vi "alicat gas monitor.vi"() -> ()   [LabVIEW 2010]
uses:
  <vilib>/Utility/file.llb/Write To Spreadsheet File (DBL).vi
panel:
  out "error out":errorcluster
  in  "Path":path
  out "Alicat gas flow monitor":cluster{dbl, dbl}[](graph)
  out "Pressure (inH2O)":dbl
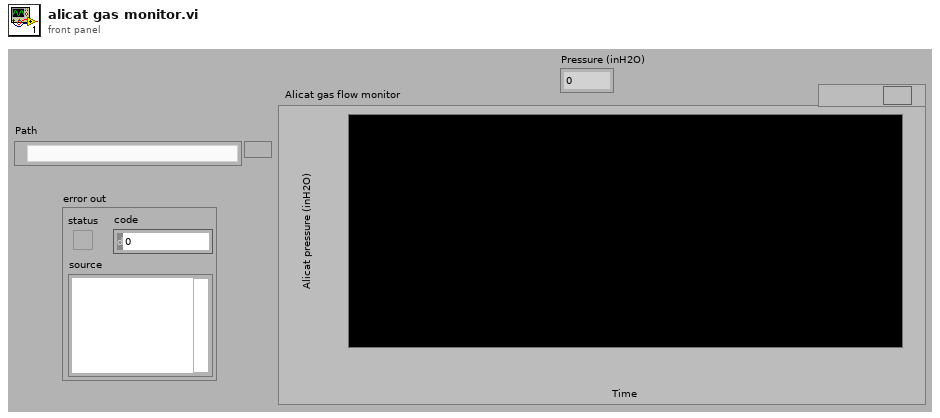
[diagram p1: front panel]
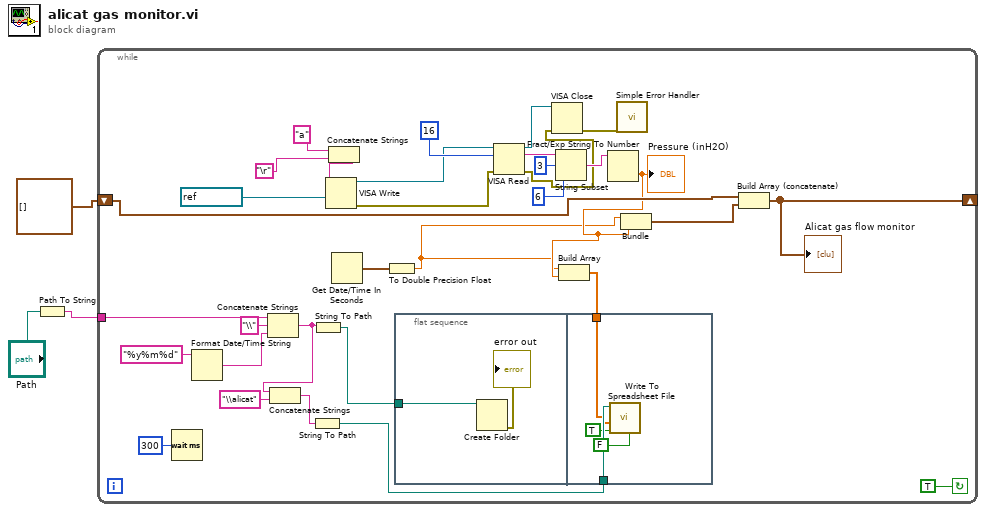
[diagram p0: block diagram]
diagram:
  n1 = Path To String(path="Path") -> (string=w1:string)
  n2 = while {
    shift-right: [w19] -> _
    shift-left: cluster{dbl, dbl}[] [] -> [w20]
    tunnel: w1 -> [w17]
    stop <- TRUE continue-if-true
    n3 = Wait (ms)(milliseconds to wait=u32 300) -> ()  [unwired: 1 out]
    n4 = Format Date/Time String(time format string (%c)="%y%m%d") -> (date/time string=w15:string)  [unwired: 2 in]
    n5 = Concatenate Strings(w17, "\\" ("string"), w15) -> (w12:string)
    n6 = Concatenate Strings(w12, "\\alicat" ("string")) -> (w11:string)
    n7 = String To Path(string=w11) -> (path=w10:path)
    n8 = String To Path(string=w12) -> (path=w14:path)
    n9 = Concatenate Strings("a" ("string"), "\r") -> (w34:string)
    n10 = VISA Write(VISA resource name=refnum<visa-resource-name> "COM6", write buffer=w34) -> (VISA resource name out=w29:refnum<visa-resource-name>, error out=w30:errorcluster)  [unwired: 1 in, 1 out]
    n11 = Get Date/Time In Seconds() -> (seconds since 1Jan1904=w22:timestamp)
    n12 = To Double Precision Float(number=w22) -> (double precision float=w8:dbl)
    n13 = flat-sequence {
      tunnel: w14 -> [w37]
      tunnel: w10 -> [w41]
      tunnel: w7 -> [w38]
      frame #0 {
        n14 = Create Folder(path (use dialog)=w37) -> (error out=→"error out":errorcluster)  [unwired: 2 in, 2 out]
      }
      frame #1 {
        n15 = call-poly <vilib>:"Write To Spreadsheet File.vi"("transpose? (no:F)"=FALSE, "append to file? (new file:F)"=TRUE, "1D data"=w38, "file path (dialog if empty)"=w41) -> ()  [unwired: 4 in, 1 out]
      }
    }
    n16 = VISA Read(VISA resource name=w29, byte count=u32 16 ("bytes to read 2"), error in (no error)=w30) -> (VISA resource name out=w5:refnum<visa-resource-name>, read buffer=w28:string, error out=w4:errorcluster)  [unwired: 1 out]
    n17 = VISA Close(VISA resource name=w5, error in (no error)=w4) -> (error out=w6:errorcluster)
    n18 = String Subset(string=w28, offset (0)=3, length (rest)=6 ("length (rest)")) -> (substring=w25:string)
    n19 = Fract/Exp String To Number(string=w25) -> (number=w9:dbl)  [unwired: 3 in, 1 out]
    "Pressure (inH2O)" <- w9
    n20 = Build Array(w8, w9) -> (w7:dbl[])
    n21 = call <vilib>:"Simple Error Handler.vi"("error in (no error)"=w6) -> ()  [unwired: 4 in, 5 out]
    n22 = Bundle(w8, w9) -> (w21:cluster{dbl, dbl})  [unwired: 1 in]
    n23 = Build Array (concatenate)(w20, w21) -> (w19:cluster{dbl, dbl}[])
    "Alicat gas flow monitor" <- w19
  }
